vi "Run.vi"(7 "Team Index":i32, 8 "Column":i32, 9 "Row":i32, 10 "View":i32[](array[numeric]) caption="View (Team Index, -1: empty)", 11 "Runner in":refnum<class "Sentinel.lvclass">) -> (0 "Replicated":refnum<class "Square.lvclass">, 1 "Direction":T1, 2 "Action":T2, 3 "Runner out":refnum<class "Sentinel.lvclass">)   [LabVIEW 2015, in "Sentinel.lvclass"]
uses:
  Sentinel.lvclass
  Type Defs/Action Enum.ctl
  Type Defs/Direction Enum.ctl
  Square/Square.lvclass
  Common/Attack Options.ctl
  Sentinel.lvclass/Sentinel.ctl
  SubVIs/Read-Only Globals.vi
  Common/Find Enemy.vi
  Common/Reverse Direction.vi
  SubVIs/Globals (private).vi
  Type Defs/SB Type Defs.lvlib
  Common/Common.lvlib
panel:
  # "NW\nN\nNE\nE\nSE\nS\nSW\nW"
  # "NOTICE - YOU MUST NOT REMOVE THIS NOTICE. PER THE FOLLOWING LICENSE, YOU MAY REPRODUCE THIS SOFTWARE PROVIDED YOU FOLLOW THE TERMS\nOF THE LICENSE.\n\n---BEGIN BSD LICENSE (http://opensource.org/licenses/BSD-2-Clause)---\nCopyright (c) 2015, Endigit, Inc. <robert@endigit.com>\nAll rights reserved.\n\nRedistribution and use in source and binary forms, with or without modification, are permitted provided that the following conditions are met:\n\n1. Redistributions of source code must retain the above copyright notice, this list of conditions and the following disclaimer.\n\n2. Redistributions in binary form must reproduce the above copyright notice, this list of conditions and the following disclaimer in the documentation and/or other \nmaterials provided with the distribution.\n\nTHIS SOFTWARE IS PROVIDED BY THE COPYRIGHT HOLDERS AND CONTRIBUTORS \"AS IS\" AND ANY EXPRESS OR IMPLIED WARRANTIES, INCLUDING, BUT NOT \nLIMITED TO, THE IMPLIED WARRANTIES OF MERCHANTABILITY AND FITNESS FOR A PARTICULAR PURPOSE ARE DISCLAIMED. IN NO EVENT SHALL THE COPYRIGHT \nHOLDER OR CONTRIBUTORS BE LIABLE FOR ANY DIRECT, INDIRECT, INCIDENTAL, SPECIAL, EXEMPLARY, OR CONSEQUENTIAL DAMAGES (INCLUDING, BUT NOT \nLIMITED TO, PROCUREMENT OF SUBSTITUTE GOODS OR SERVICES; LOSS OF USE, DATA, OR PROFITS; OR BUSINESS INTERRUPTION) HOWEVER CAUSED AND ON \nANY THEORY OF LIABILITY, WHETHER IN CONTRACT, STRICT LIABILITY, OR TORT (INCLUDING NEGLIGENCE OR OTHERWISE) ARISING IN ANY WAY OUT OF THE USE \nOF THIS SOFTWARE, EVEN IF ADVISED OF THE POSSIBILITY OF SUCH DAMAGE.\n---END BSD LICENSE---"
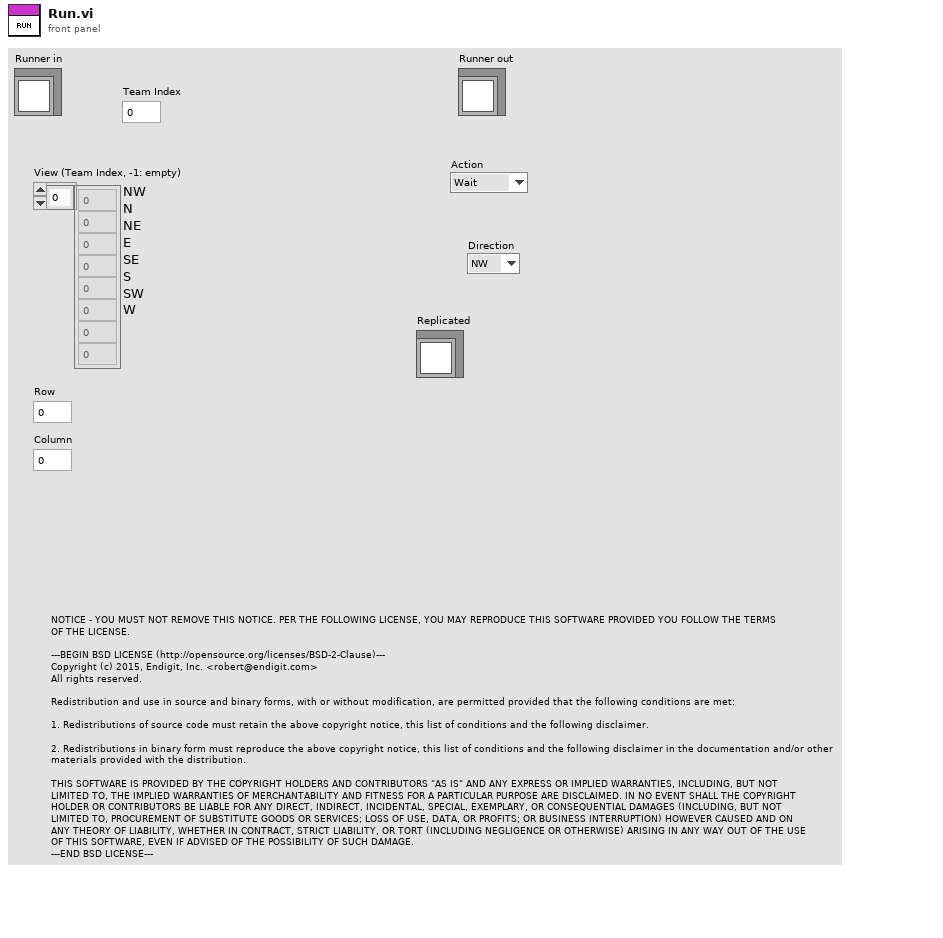
[diagram p1: front panel]
types:
  T1 = typedef "SB Type Defs.lvlib/Direction Enum.ctl" = enum16{"NW", "N", "NE", "E", "SE", "S", "SW", "W"}
  T2 = typedef "SB Type Defs.lvlib/Action Enum.ctl" = enum16{"Wait", "Move", "Attack", "Replicate"}
  T3 = typedef "Common.lvlib/Attack Options.ctl" = enum16{"Attack", "Run", "Distract"}
  T4 = enum16{"Replicator", "Replicatee", "Eastwards", "Westwards"}
  T5 = enum16{"Replication", "Northwards", "Southwards"}
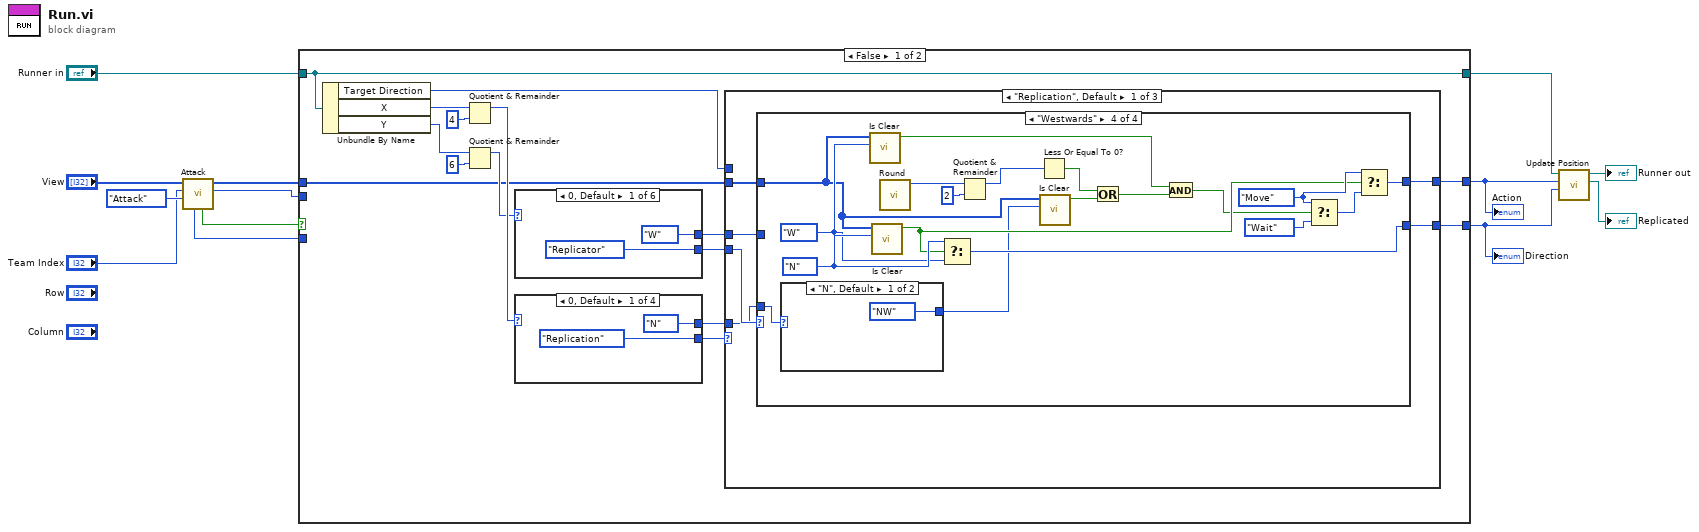
[diagram p0: block diagram]
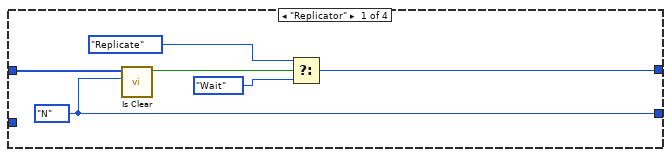
[diagram p2: hidden frame]
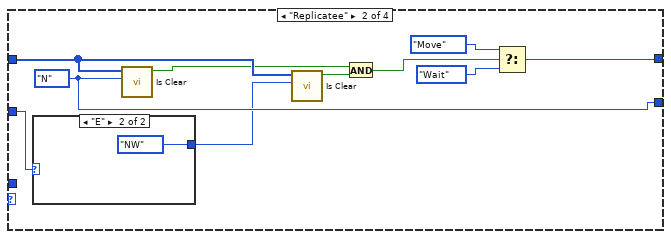
[diagram p3: hidden frame]
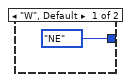
[diagram p4: hidden frame]
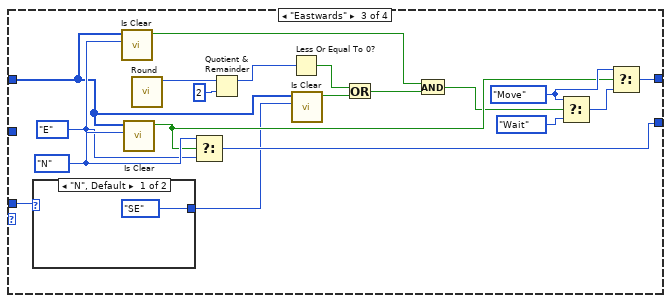
[diagram p5: hidden frame]
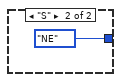
[diagram p6: hidden frame]
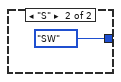
[diagram p7: hidden frame]
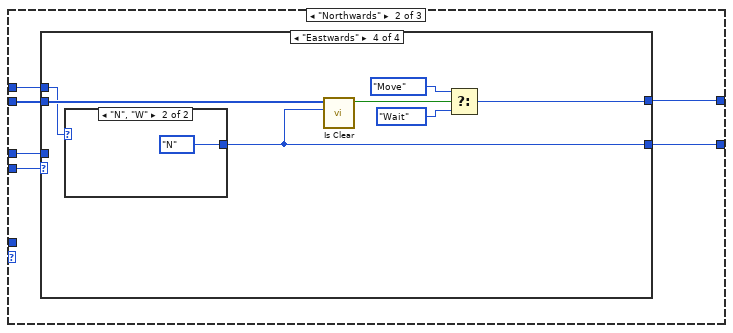
[diagram p8: hidden frame]
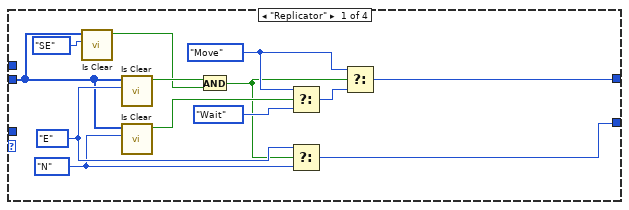
[diagram p9: hidden frame]
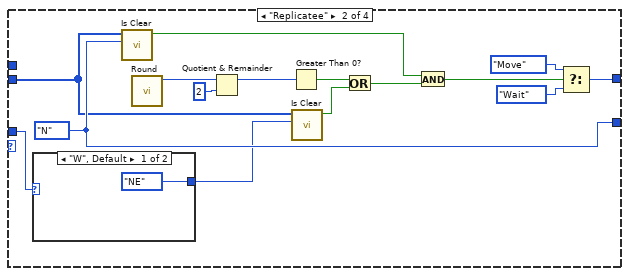
[diagram p10: hidden frame]
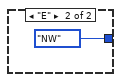
[diagram p11: hidden frame]
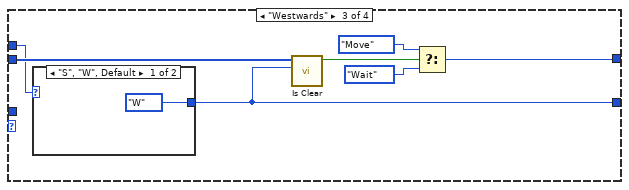
[diagram p12: hidden frame]
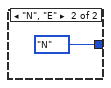
[diagram p13: hidden frame]
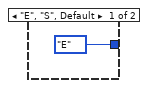
[diagram p14: hidden frame]
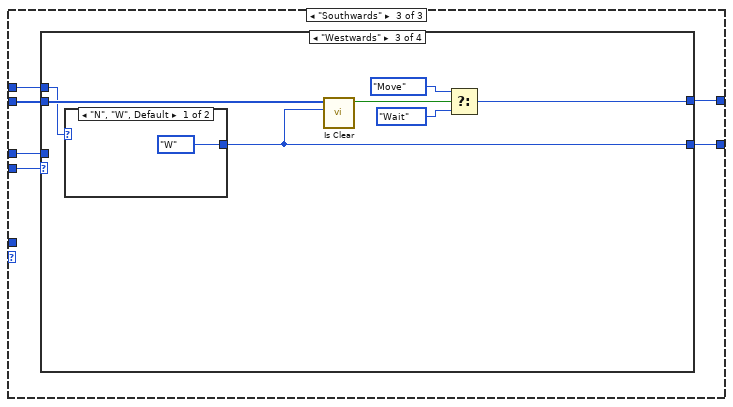
[diagram p15: hidden frame]
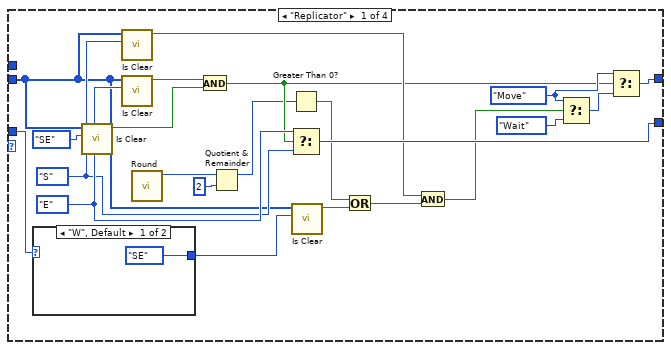
[diagram p16: hidden frame]
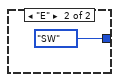
[diagram p17: hidden frame]
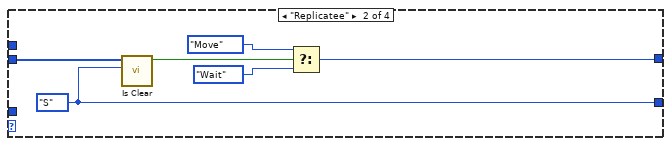
[diagram p18: hidden frame]
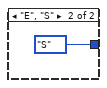
[diagram p19: hidden frame]
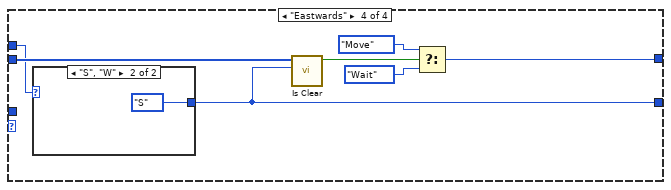
[diagram p20: hidden frame]
diagram:
  n1 = call "Attack.vi"("Attack?"=Attack_Options."Attack", "Team Index"="Team Index", "View"="View") -> ("Action"=w12:T2, "View"=w9:i32[], "Enemy Found?"=w13:bool, "Enemy Direction"=w11:i32)  [unwired: 3 in, 2 out]
  n2 = case shown="False" w13 {
    tunnel: "Runner in" -> [w20 w223]
    tunnel: w12 -> [_ w225]
    tunnel: [w19 w225] -> w3
    tunnel: w11 -> [_ w224]
    tunnel: [w18 w224] -> w4
    tunnel: [w20 w223] -> w7
    tunnel: w9 -> [w17 _]
    frame False {
      n3 = Unbundle By Name(w20) -> ("Target Direction"=w15:T1, "X"=w28:i16, "Y"=w24:i16)
      n4 = Quotient & Remainder(x=w28, y=4) -> (x-y*floor(x/y)=w26:i32)  [unwired: 1 out]
      n5 = Quotient & Remainder(x=w24, y=6) -> (x-y*floor(x/y)=w23:i32)  [unwired: 1 out]
      n6 = case shown="0, Default" w23 {
        tunnel: [T4."Replicator" ("Rows") T4."Replicatee" ("Rows") T4."Eastwards" ("Rows") T4."Replicator" ("Rows") T4."Replicatee" ("Rows") T4."Westwards" ("Rows")] -> w21
        tunnel: [Direction_Enum."W" ("Direction") Direction_Enum."E" ("Direction") Direction_Enum."E" ("Direction") Direction_Enum."E" ("Direction") Direction_Enum."W" ("Direction") Direction_Enum."W" ("Direction")] -> w16
        frame 0, Default {
        }
        frame 1 {
        }
        frame 2 {
        }
        frame 3 {
        }
        frame 4 {
        }
        frame 5 {
        }
      }
      n7 = case shown="0, Default" w26 {
        tunnel: [Direction_Enum."N" ("Direction") Direction_Enum."N" ("Direction") Direction_Enum."S" ("Direction") Direction_Enum."S" ("Direction")] -> w14
        tunnel: [T5."Replication" ("Cols") T5."Northwards" ("Cols") T5."Replication" ("Cols") T5."Southwards" ("Cols")] -> w22
        frame 0, Default {
        }
        frame 1 {
        }
        frame 2 {
        }
        frame 3 {
        }
      }
      n8 = case shown="\"Replication\", Default" w22 {
        tunnel: w21 -> [w34 w100 w154]
        tunnel: [w33 w99 w153] -> w19
        tunnel: [w32 w98 w152] -> w18
        tunnel: w17 -> [w31 w97 w151]
        tunnel: w16 -> [w30 w96 w150]
        tunnel: w15 -> [_ w95 w149]
        tunnel: w14 -> [w29 _ _]
        frame "Replication", Default {
          n9 = case shown="\"Westwards\"" w34 {
            tunnel: [w37 w47 w71 w92] -> w33
            tunnel: [w39 w50 w68 w89] -> w32
            tunnel: w31 -> [w40 w45 w54 w79]
            tunnel: w30 -> [_ w46 _ _]
            tunnel: w29 -> [_ _ w53 w74]
            frame "Replicator" {
              w39 = Direction_Enum."N" ("Direction")
              n10 = call "Is Clear.vi"("Direction"=w39, "Maze (0: Empty, -1: Enemy. >0: Teammate in"=w40) -> ("Is Clear"=w35:bool)  [unwired: 9 in]
              n11 = Select(t=Action_Enum."Replicate" ("Action"), s=w35, f=Action_Enum."Wait" ("Action")) -> (s? t:f=w37:T2)
            }
            frame "Replicatee" {
              w50 = Direction_Enum."N" ("Direction")
              n12 = case shown="\"E\"" w46 {
                tunnel: [Direction_Enum."NE" ("Direction") Direction_Enum."NW" ("Direction")] -> w44
                frame "W", Default {
                }
                frame "E" {
                }
              }
              n13 = call "Is Clear.vi"("Direction"=w50, "Maze (0: Empty, -1: Enemy. >0: Teammate in"=w45) -> ("Is Clear"=w42:bool)  [unwired: 9 in]
              n14 = call "Is Clear.vi"("Direction"=w44, "Maze (0: Empty, -1: Enemy. >0: Teammate in"=w45) -> ("Is Clear"=w43:bool)  [unwired: 9 in]
              n15 = And(x=w42, y=w43) -> (x .and. y?=w41:bool)
              n16 = Select(t=Action_Enum."Move" ("Action"), s=w41, f=Action_Enum."Wait" ("Action")) -> (s? t:f=w47:T2)
            }
            frame "Eastwards" {
              w69 = Direction_Enum."E" ("Direction")
              w66 = Action_Enum."Move" ("Action")
              w70 = Direction_Enum."N" ("Direction")
              n17 = case shown="\"N\", Default" w53 {
                tunnel: [Direction_Enum."SE" ("Direction") Direction_Enum."NE" ("Direction")] -> w59
                frame "N", Default {
                }
                frame "S" {
                }
              }
              n18 = call "Is Clear.vi"("Direction"=w69, "Maze (0: Empty, -1: Enemy. >0: Teammate in"=w54) -> ("Is Clear"=w58:bool)  [unwired: 9 in]
              n19 = call "Is Clear.vi"("Direction"=w70, "Maze (0: Empty, -1: Enemy. >0: Teammate in"=w54) -> ("Is Clear"=w64:bool)  [unwired: 9 in]
              n20 = call "Round.vi"() -> ("Round"=w63:i32)  [unwired: 11 in]
              n21 = Select(t=w70, s=w64, f=w69) -> (s? t:f=w68:T1)
              n22 = Quotient & Remainder(x=w63, y=2) -> (x-y*floor(x/y)=w61:i32)  [unwired: 1 out]
              n23 = Less Or Equal To 0?(x=w61) -> (x <= 0?=w60:bool)
              n24 = call "Is Clear.vi"("Direction"=w59, "Maze (0: Empty, -1: Enemy. >0: Teammate in"=w54) -> ("Is Clear"=w57:bool)  [unwired: 9 in]
              n25 = Or(x=w60, y=w57) -> (x .or. y?=w56:bool)
              n26 = And(x=w58, y=w56) -> (x .and. y?=w55:bool)
              n27 = Select(t=w66, s=w55, f=Action_Enum."Wait" ("Action")) -> (s? t:f=w65:T2)
              n28 = Select(t=w66, s=w64, f=w65) -> (s? t:f=w71:T2)
            }
            frame "Westwards" {
              w90 = Direction_Enum."W" ("Direction")
              w87 = Action_Enum."Move" ("Action")
              w91 = Direction_Enum."N" ("Direction")
              n29 = case shown="\"N\", Default" w74 {
                tunnel: [Direction_Enum."NW" ("Direction") Direction_Enum."SW" ("Direction")] -> w80
                frame "N", Default {
                }
                frame "S" {
                }
              }
              n30 = call "Is Clear.vi"("Direction"=w90, "Maze (0: Empty, -1: Enemy. >0: Teammate in"=w79) -> ("Is Clear"=w78:bool)  [unwired: 9 in]
              n31 = call "Is Clear.vi"("Direction"=w91, "Maze (0: Empty, -1: Enemy. >0: Teammate in"=w79) -> ("Is Clear"=w85:bool)  [unwired: 9 in]
              n32 = call "Round.vi"() -> ("Round"=w83:i32)  [unwired: 11 in]
              n33 = Select(t=w91, s=w85, f=w90) -> (s? t:f=w89:T1)
              n34 = Quotient & Remainder(x=w83, y=2) -> (x-y*floor(x/y)=w82:i32)  [unwired: 1 out]
              n35 = Less Or Equal To 0?(x=w82) -> (x <= 0?=w81:bool)
              n36 = call "Is Clear.vi"("Direction"=w80, "Maze (0: Empty, -1: Enemy. >0: Teammate in"=w79) -> ("Is Clear"=w77:bool)  [unwired: 9 in]
              n37 = Or(x=w81, y=w77) -> (x .or. y?=w76:bool)
              n38 = And(x=w78, y=w76) -> (x .and. y?=w75:bool)
              n39 = Select(t=w87, s=w75, f=Action_Enum."Wait" ("Action")) -> (s? t:f=w86:T2)
              n40 = Select(t=w87, s=w85, f=w86) -> (s? t:f=w92:T2)
            }
          }
        }
        frame "Northwards" {
          n41 = case shown="\"Eastwards\"" w100 {
            tunnel: [w108 w125 w134 w143] -> w99
            tunnel: [w109 w126 w131 w140] -> w98
            tunnel: w97 -> [w107 w124 w133 w142]
            tunnel: w96 -> [_ w122 _ _]
            tunnel: w95 -> [_ _ w132 w141]
            frame "Replicator" {
              w102 = Direction_Enum."N" ("Direction")
              w110 = Direction_Enum."E" ("Direction")
              w105 = Action_Enum."Move" ("Action")
              n42 = call "Is Clear.vi"("Direction"=Direction_Enum."SE", "Maze (0: Empty, -1: Enemy. >0: Teammate in"=w107) -> ("Is Clear"=w111:bool)  [unwired: 9 in]
              n43 = call "Is Clear.vi"("Direction"=w110, "Maze (0: Empty, -1: Enemy. >0: Teammate in"=w107) -> ("Is Clear"=w112:bool)  [unwired: 9 in]
              n44 = call "Is Clear.vi"("Direction"=w102, "Maze (0: Empty, -1: Enemy. >0: Teammate in"=w107) -> ("Is Clear"=w104:bool)  [unwired: 9 in]
              n45 = And(x=w112, y=w111) -> (x .and. y?=w101:bool)
              n46 = Select(t=w105, s=w104, f=Action_Enum."Wait" ("Action")) -> (s? t:f=w103:T2)
              n47 = Select(t=w110, s=w101, f=w102) -> (s? t:f=w109:T1)
              n48 = Select(t=w105, s=w101, f=w103) -> (s? t:f=w108:T2)
            }
            frame "Replicatee" {
              w126 = Direction_Enum."N" ("Direction")
              n49 = case shown="\"W\", Default" w122 {
                tunnel: [Direction_Enum."NE" ("Direction") Direction_Enum."NW" ("Direction")] -> w121
                frame "W", Default {
                }
                frame "E" {
                }
              }
              n50 = call "Is Clear.vi"("Direction"=w126, "Maze (0: Empty, -1: Enemy. >0: Teammate in"=w124) -> ("Is Clear"=w123:bool)  [unwired: 9 in]
              n51 = call "Round.vi"() -> ("Round"=w119:i32)  [unwired: 11 in]
              n52 = Quotient & Remainder(x=w119, y=2) -> (x-y*floor(x/y)=w116:i32)  [unwired: 1 out]
              n53 = Greater Than 0?(x=w116) -> (x > 0?=w115:bool)
              n54 = call "Is Clear.vi"("Direction"=w121, "Maze (0: Empty, -1: Enemy. >0: Teammate in"=w124) -> ("Is Clear"=w117:bool)  [unwired: 9 in]
              n55 = Or(x=w115, y=w117) -> (x .or. y?=w114:bool)
              n56 = And(x=w123, y=w114) -> (x .and. y?=w120:bool)
              n57 = Select(t=Action_Enum."Move" ("Action"), s=w120, f=Action_Enum."Wait" ("Action")) -> (s? t:f=w125:T2)
            }
            frame "Westwards" {
              n58 = case shown="\"S\", \"W\", Default" w132 {
                tunnel: [Direction_Enum."W" ("Direction") Direction_Enum."N" ("Direction")] -> w131
                frame "S", "W", Default {
                }
                frame "N", "E" {
                }
              }
              n59 = call "Is Clear.vi"("Direction"=w131, "Maze (0: Empty, -1: Enemy. >0: Teammate in"=w133) -> ("Is Clear"=w135:bool)  [unwired: 9 in]
              n60 = Select(t=Action_Enum."Move" ("Action"), s=w135, f=Action_Enum."Wait" ("Action")) -> (s? t:f=w134:T2)
            }
            frame "Eastwards" {
              n61 = case shown="\"N\", \"W\"" w141 {
                tunnel: [Direction_Enum."E" ("Direction") Direction_Enum."N" ("Direction")] -> w140
                frame "E", "S", Default {
                }
                frame "N", "W" {
                }
              }
              n62 = call "Is Clear.vi"("Direction"=w140, "Maze (0: Empty, -1: Enemy. >0: Teammate in"=w142) -> ("Is Clear"=w144:bool)  [unwired: 9 in]
              n63 = Select(t=Action_Enum."Move" ("Action"), s=w144, f=Action_Enum."Wait" ("Action")) -> (s? t:f=w143:T2)
            }
          }
        }
        frame "Southwards" {
          n64 = case shown="\"Westwards\"" w154 {
            tunnel: [w171 w181 w188 w197] -> w153
            tunnel: [w172 w182 w185 w194] -> w152
            tunnel: w151 -> [w166 w180 w187 w196]
            tunnel: w150 -> [w163 _ _ _]
            tunnel: w149 -> [_ _ w186 w195]
            frame "Replicator" {
              w167 = Direction_Enum."S" ("Direction")
              w173 = Direction_Enum."E" ("Direction")
              w169 = Action_Enum."Move" ("Action")
              n65 = case shown="\"W\", Default" w163 {
                tunnel: [Direction_Enum."SE" ("Direction") Direction_Enum."SW" ("Direction")] -> w162
                frame "W", Default {
                }
                frame "E" {
                }
              }
              n66 = call "Is Clear.vi"("Direction"=Direction_Enum."SE", "Maze (0: Empty, -1: Enemy. >0: Teammate in"=w166) -> ("Is Clear"=w174:bool)  [unwired: 9 in]
              n67 = call "Is Clear.vi"("Direction"=w167, "Maze (0: Empty, -1: Enemy. >0: Teammate in"=w166) -> ("Is Clear"=w165:bool)  [unwired: 9 in]
              n68 = call "Is Clear.vi"("Direction"=w173, "Maze (0: Empty, -1: Enemy. >0: Teammate in"=w166) -> ("Is Clear"=w175:bool)  [unwired: 9 in]
              n69 = call "Round.vi"() -> ("Round"=w157:i32)  [unwired: 11 in]
              n70 = And(x=w175, y=w174) -> (x .and. y?=w161:bool)
              n71 = Quotient & Remainder(x=w157, y=2) -> (x-y*floor(x/y)=w159:i32)  [unwired: 1 out]
              n72 = Greater Than 0?(x=w159) -> (x > 0?=w160:bool)
              n73 = Select(t=w173, s=w161, f=w167) -> (s? t:f=w172:T1)
              n74 = call "Is Clear.vi"("Direction"=w162, "Maze (0: Empty, -1: Enemy. >0: Teammate in"=w166) -> ("Is Clear"=w156:bool)  [unwired: 9 in]
              n75 = Or(x=w160, y=w156) -> (x .or. y?=w155:bool)
              n76 = And(x=w165, y=w155) -> (x .and. y?=w164:bool)
              n77 = Select(t=w169, s=w164, f=Action_Enum."Wait" ("Action")) -> (s? t:f=w168:T2)
              n78 = Select(t=w169, s=w161, f=w168) -> (s? t:f=w171:T2)
            }
            frame "Replicatee" {
              w182 = Direction_Enum."S" ("Direction")
              n79 = call "Is Clear.vi"("Direction"=w182, "Maze (0: Empty, -1: Enemy. >0: Teammate in"=w180) -> ("Is Clear"=w179:bool)  [unwired: 9 in]
              n80 = Select(t=Action_Enum."Move" ("Action"), s=w179, f=Action_Enum."Wait" ("Action")) -> (s? t:f=w181:T2)
            }
            frame "Westwards" {
              n81 = case shown="\"N\", \"W\", Default" w186 {
                tunnel: [Direction_Enum."W" ("Direction") Direction_Enum."S" ("Direction")] -> w185
                frame "N", "W", Default {
                }
                frame "E", "S" {
                }
              }
              n82 = call "Is Clear.vi"("Direction"=w185, "Maze (0: Empty, -1: Enemy. >0: Teammate in"=w187) -> ("Is Clear"=w189:bool)  [unwired: 9 in]
              n83 = Select(t=Action_Enum."Move" ("Action"), s=w189, f=Action_Enum."Wait" ("Action")) -> (s? t:f=w188:T2)
            }
            frame "Eastwards" {
              n84 = case shown="\"S\", \"W\"" w195 {
                tunnel: [Direction_Enum."E" ("Direction") Direction_Enum."S" ("Direction")] -> w194
                frame "N", "E", Default {
                }
                frame "S", "W" {
                }
              }
              n85 = call "Is Clear.vi"("Direction"=w194, "Maze (0: Empty, -1: Enemy. >0: Teammate in"=w196) -> ("Is Clear"=w198:bool)  [unwired: 9 in]
              n86 = Select(t=Action_Enum."Move" ("Action"), s=w198, f=Action_Enum."Wait" ("Action")) -> (s? t:f=w197:T2)
            }
          }
        }
      }
    }
    frame True {
    }
  }
  "Action" <- w3
  "Direction" <- w4
  n87 = call-dynamic "Update Position.vi"("Direction"=w4, "Action"=w3, "Sentinel in"=w7) -> ("Sentinel in 2"=→"Replicated":refnum<class "Sentinel.lvclass">, "Sentinel out"=→"Runner out":refnum<class "Sentinel.lvclass">)  [unwired: 6 in, 1 out]
